vi "Read Device Address.vi"(11 "PIC-Device in":refnum<class "PIC-Device.lvclass">) -> (2 "Device Address":u8=6 min=6 max=7 step=1, 3 "PIC-Device out":refnum<class "PIC-Device.lvclass">)   [LabVIEW 2020, in "PIC-Device.lvclass"]
uses:
  PIC-Device.lvclass
  PIC-Device.lvclass/PIC-Device.ctl
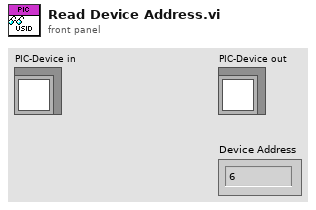
[diagram p1: front panel]
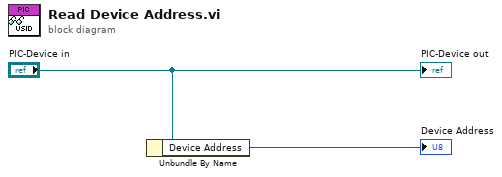
[diagram p0: block diagram]
diagram:
  n1 = Unbundle By Name("PIC-Device in") -> ("Device Address"=→"Device Address":u8)
  "PIC-Device out" <- "PIC-Device in"
